vi "BallTubeSystem.vi"(7 "error in (no error)":errorcluster, 10 "Tube up one Increment":bool) -> (0 "error out":errorcluster)   [LabVIEW 2019]
panel:
  out "End":bool
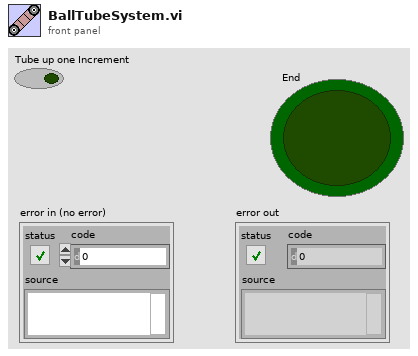
[diagram p1: front panel]
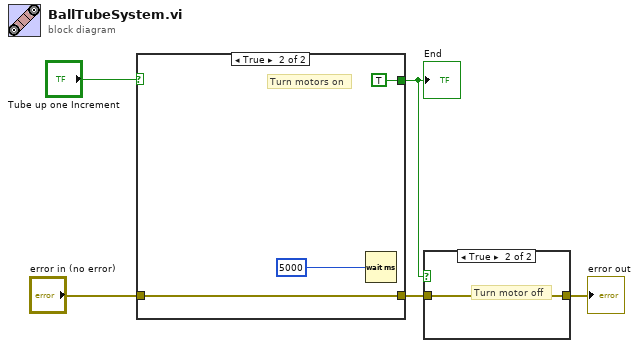
[diagram p0: block diagram]
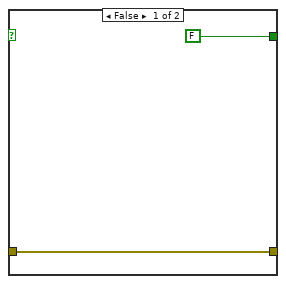
[diagram p3: hidden frame]
diagram:
  n1 = case shown="True" "Tube up one Increment" {
    tunnel: [FALSE ("Boolean") TRUE ("Boolean")] -> w5
    tunnel: [w6 w8] -> w3
    tunnel: "error in (no error)" -> [w6 w8]
    frame False {
    }
    frame True {
      # "Turn motors on"
      n2 = Wait (ms)(milliseconds to wait=u32 5000) -> ()  [unwired: 1 out]
    }
  }
  "End" <- w5
  n3 = case shown="True" w5 {
    tunnel: [w11 w12] -> w4
    tunnel: w3 -> [w11 w12]
    frame False {
    }
    frame True {
      # "Turn motor off"
    }
  }
  "error out" <- w4
